vi "Logger.vi"(7 "Custom Device Name":string, 8 "error in":errorcluster, 9 "Log":T1={"Message"="", "Level"=enum."Error", "Add to log file? (F)"=FALSE, "Append newline? (T)"=TRUE}, 10 "State":enum16{"Initialize", "Log"}(ring), 11 "Custom Device in":refnum<class "SystemMonitor Engine.lvclass">) -> (0 "error out":errorcluster, 3 "Custom Device out":refnum<class "SystemMonitor Engine.lvclass">)   [LabVIEW 2026, in "SystemMonitor Engine.lvlib" / "SystemMonitor Engine.lvclass"]
uses:
  SystemMonitor Engine.lvclass
  SystemMonitor Engine.lvclass/SystemMonitor Engine.ctl
  <userlib>/Custom Device Interfaces_v1.lvlibp/CustomDeviceAPI/Custom Device API.lvclass
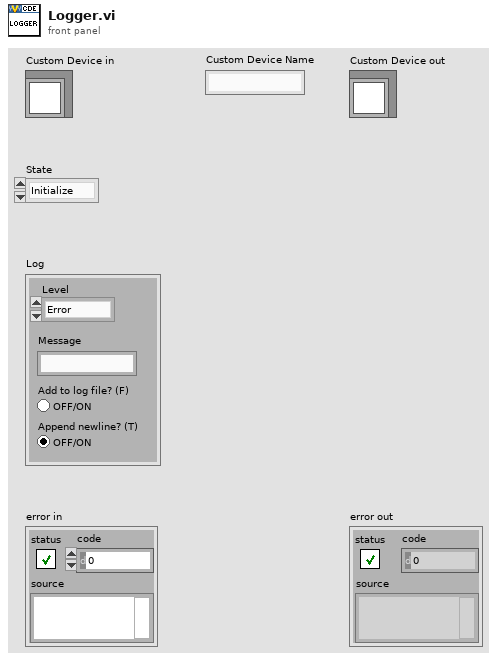
[diagram p1: front panel]
types:
  T1 = cluster{"Message":string, "Level":enum16{"Error", "Warning", "Info", "Debug"}, "Add to log file? (F)":bool, "Append newline? (T)":bool}
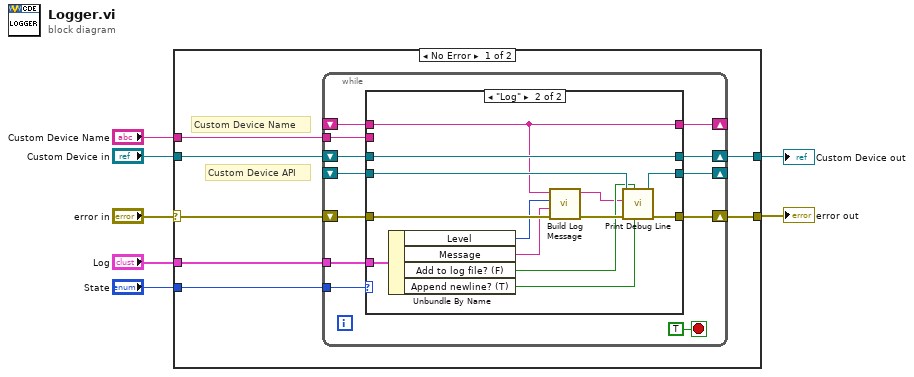
[diagram p0: block diagram]
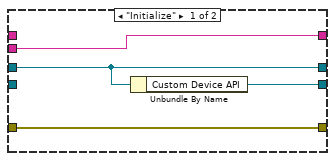
[diagram p2: hidden frame]
diagram:
  n1 = case shown="No Error" "error in" {
    selector: "error in" -> [w14 w45]
    tunnel: "Custom Device in" -> [w12 w44]
    tunnel: [w11 w44] -> w4
    tunnel: "State" -> [w10 _]
    tunnel: [w13 w45] -> w6
    tunnel: "Log" -> [w9 _]
    tunnel: "Custom Device Name" -> [w8 _]
    frame No Error {
      # "Custom Device API"
      # "Custom Device Name"
      n2 = while {
        shift-right: [w23] -> w11
        shift-left: w12 -> [w20]
        tunnel: w10 -> [w24]
        shift-right: [w22] -> _
        shift-left: _ -> [w21]
        shift-right: [w25] -> w13
        shift-left: w14 -> [w26]
        tunnel: w9 -> [w19]
        tunnel: w8 -> [w18]
        shift-right: [w17] -> _
        shift-left: _ -> [w16]
        stop <- TRUE stop-if-true
        n3 = case shown="\"Log\"" w24 {
          tunnel: w20 -> [w28 w40]
          tunnel: [w28 w40] -> w23
          tunnel: [w29 w31] -> w22
          tunnel: w21 -> [_ w39]
          tunnel: w26 -> [w30 w42]
          tunnel: [w30 w43] -> w25
          tunnel: w19 -> [_ w38]
          tunnel: w18 -> [w27 _]
          tunnel: [w27 w32] -> w17
          tunnel: w16 -> [_ w32]
          frame "Initialize" {
            n4 = Unbundle By Name(w28) -> ("Custom Device API"=w29:refnum<class "Custom Device API.lvclass">)
          }
          frame "Log" {
            n5 = Unbundle By Name(w38) -> ("Level"=w34:enum16{"Error", "Warning", "Info", "Debug"}, "Message"=w33:string, "Add to log file? (F)"=w37:bool, "Append newline? (T)"=w36:bool)
            n6 = call "Build Log Message.vi"("error in"=w42, "Message"=w33, "Level"=w34, "Custom Device Name"=w32) -> ("error out"=w41:errorcluster, "Log Message"=w35:string)  [unwired: 6 in]
            n7 = call-dynamic "Print Debug Line.vi"("Append newline? (T)"=w36, "Add to log file? (F)"=w37, "error in"=w41, "Message"=w35, "Custom Device API in"=w39) -> ("error out"=w43:errorcluster, "Custom Device API out"=w31:refnum<class "Custom Device API.lvclass">)  [unwired: 5 in]
          }
        }
      }
    }
    frame Error {
    }
  }
  "Custom Device out" <- w4
  "error out" <- w6
